vi "Check Crossing A Valve.vi"(1 "Logic Cluster":T1, 2 "Valve Open?":bool, 3 "Target Pos":dbl, 4 "Current Pos":dbl) -> (0 "Crossing Valve Error":bool)   [LabVIEW 2016, in "Hardware.lvlib" / "VacuumLine.lvlib" / "VacuumLine.lvclass"]
uses:
  <userlib>/Common Components/Hardware/Abstract System/VacuumLine/VacuumLine/VacuumLine.lvclass
  <userlib>/Common Components/Hardware/Abstract System/VacuumLine/VacuumLine/Logic Cluster.ctl
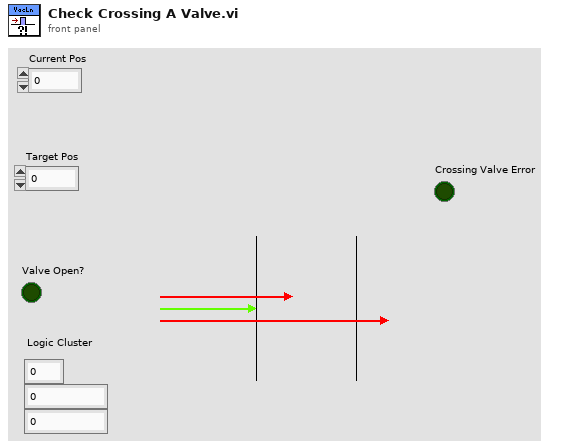
[diagram p1: front panel]
types:
  T1 = typedef "Hardware.lvlib/VacuumLine.lvlib/VacuumLine.lvclass/Logic Cluster.ctl" = cluster{"Pin#":u8, "Location":dbl, "Tolerance":dbl}
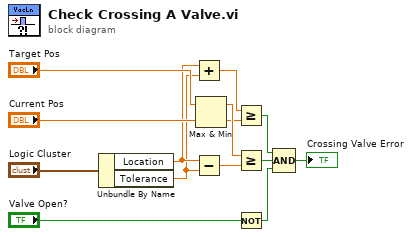
[diagram p0: block diagram]
diagram:
  n1 = Unbundle By Name("Logic Cluster") -> ("Location"=w8:dbl, "Tolerance"=w7:dbl)
  n2 = Add(x=w8, y=w7) -> (x+y=w5:dbl)
  n3 = Subtract(x=w8, y=w7) -> (x-y=w3:dbl)
  n4 = Max & Min(x="Target Pos", y="Current Pos") -> (max(x,y)=w6:dbl, min(x,y)=w4:dbl)
  n5 = Greater Or Equal?(x=w5, y=w4) -> (x >= y?=w2:bool)
  n6 = Greater Or Equal?(x=w6, y=w3) -> (x >= y?=w1:bool)
  n7 = Not(x="Valve Open?") -> (.not. x?=w12:bool)
  n8 = Compound Arithmetic op=AND(w2, w1, w12) -> (→"Crossing Valve Error":bool)
